vi "SearchAndReplaceJitEx.vi"(4 "Options":u32 format="%.0x", 5 "replace all? (F)":bool, 6 "offset":i32, 7 "substring to replace":i32, 8 "error in":errorcluster, 9 "replace string":string, 10 "search pattern":string, 11 "string":string) -> (0 "error out":errorcluster, 1 "offset past replacement":i32, 2 "number of replacements":i32, 3 "string":string)   [LabVIEW 2021, in "libpcre2-8.lvlib"]
uses:
  libpcre2-8.lvlib
  Pcre2GetOvectorPointer8.vi
  Pcre2MoOfSubstrNumFmOv.vi
  Pcre2SubstringFromSubjectByOffsets (s).vi
  Pcre2CompileError.vi
  Pcre2FnkCallError.vi
  Pcre2ErrorNull.vi
  Pcre2LibError.vi
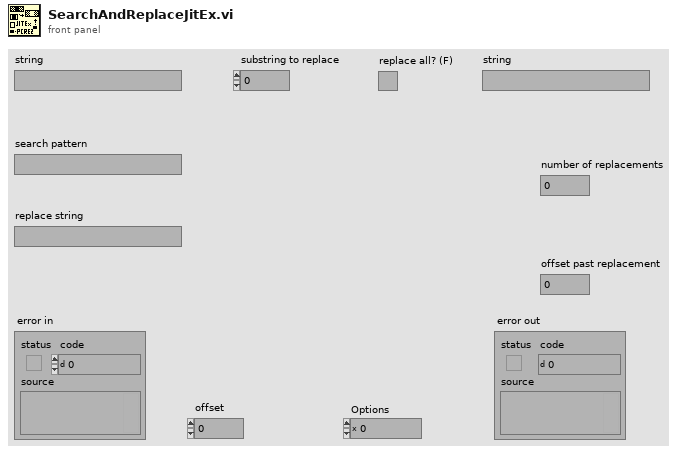
[diagram p1: front panel]
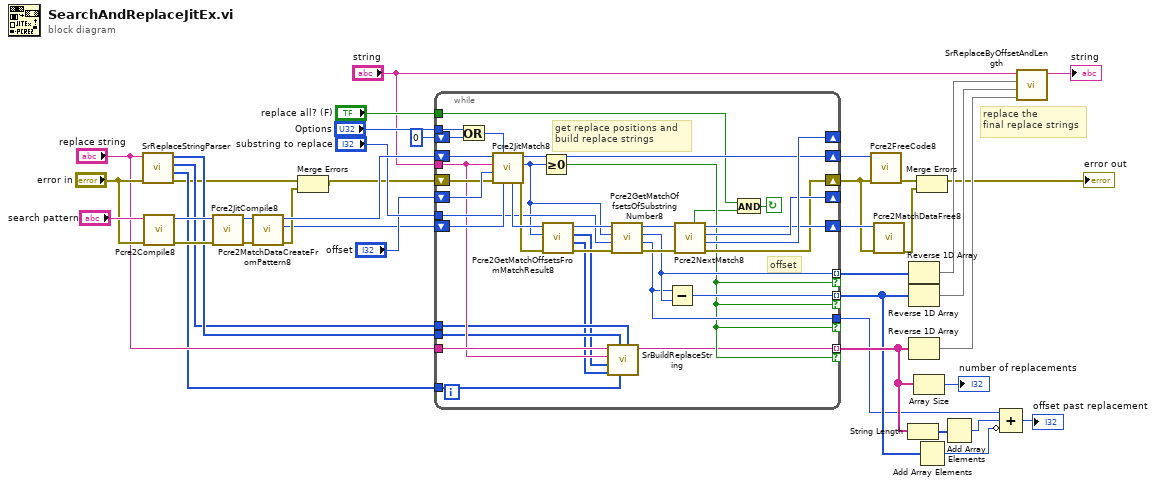
[diagram p0: block diagram]
diagram:
  # "replace the \nfinal replace strings"
  n1 = call "SrReplaceStringParser.vi"("error in"="error in", "ReplaceString"="replace string") -> ("error out"=w5:errorcluster, "ReplSubStrNum"=w14:i32[], "ReplStrLengths"=w15:i32[], "ReplStrOffsets"=w16:i32[])  [unwired: 6 in]
  n2 = call "Pcre2Compile8.vi"("error in"="error in", "Pattern"="search pattern") -> ("error out"=w37:errorcluster, "pCode"=w36:u64)  [unwired: 8 in]
  n3 = call "Pcre2JitCompile8.vi"("error in"=w37, "pCode"=w36) -> ("error out"=w40:errorcluster, "pCode"=w38:u64)  [unwired: 8 in]
  n4 = call "Pcre2MatchDataCreateFromPattern8.vi"("error in"=w40, "pCode"=w38) -> ("error out"=w4:errorcluster, "pMatchData"=w1:u64, "pCode"=w39:u64)  [unwired: 7 in]
  n5 = Merge Errors(w5, w4) -> (w3:errorcluster)
  n6 = while {
    tunnel: "string" -> [w47]
    shift-right: [w71] -> _
    shift-left: "offset" -> [w74]
    shift-right: [w69] -> w32
    shift-left: w1 -> [w73]
    shift-right: [w72] -> _
    shift-left: u32 0 ("GlobalOptions") -> [w56]
    shift-right: [w70] -> w33
    shift-left: w39 -> [w75]
    shift-right: [w67] -> w31
    shift-left: w3 -> [w68]
    tunnel: "replace string" -> [w48]
    tunnel: "substring to replace" -> [w63]
    tunnel: [w41] -> w26 mode=indexing if=w52
    tunnel: [w59] -> w25 mode=indexing if=w52
    tunnel: [w58] -> w34 mode=indexing if=w52
    tunnel: "Options" -> [w54]
    tunnel: [w53] -> w23 if=w52
    tunnel: "replace all? (F)" -> [w51]
    tunnel: w16 -> [w46]
    tunnel: w15 -> [w45]
    tunnel: w14 -> [w44]
    stop <- w49 continue-if-true
    # "get replace positions and \nbuild replace strings"
    # "offset"
    n7 = Or(x=w54, y=w56) -> (x .or. y?=w55:u32)
    n8 = call "Pcre2JitMatch8.vi"("pMatchData"=w73, "Options"=w55, "error in"=w68, "StartOffset"=w74, "Subject"=w47, "pCode"=w75) -> ("error out"=w65:errorcluster, "MatchResult"=w60:i32, "pCode"=w70:u64, "pMatchData"=w66:u64)  [unwired: 2 in]
    n9 = Greater Or Equal To 0?(x=w60) -> (x >= 0?=w52:bool)
    n10 = call "Pcre2GetMatchOffsetsFromMatchResult8.vi"("error in"=w65, "MatchResult"=w60, "pMatchData"=w66) -> ("error out"=w57:errorcluster, "OffsetsPastMatch"=w43:i32[], "MatchOffsets"=w42:i32[], "pMatchData"=w64:u64)  [unwired: 5 in]
    n11 = call "SrBuildReplaceString.vi"("ReplStrLengths"=w45, "ReplSubStrNum"=w44, "ReplStrOffsets"=w46, "OffsetsPastMatch"=w43, "MatchOffsets"=w42, "Subject"=w47, "ReplaceString"=w48) -> ("ReplaceString"=w41:string)  [unwired: 4 in]
    n12 = call "Pcre2GetMatchOffsetsOfSubstringNumber8.vi"("error in"=w57, "Number"=w63, "MatchResult"=w60, "pMatchData"=w64) -> ("error out"=w61:errorcluster, "OffsetPastMatch"=w53:i32, "MatchOffset"=w58:i32, "pMatchData"=w62:u64)  [unwired: 4 in]
    n13 = Subtract(x=w53, y=w58) -> (x-y=w59:i32)
    n14 = call "Pcre2NextMatch8.vi"("error in"=w61, "pMatchData"=w62) -> ("error out"=w67:errorcluster, "GlobalOptions"=w72:u32, "NextStartOffset"=w71:u64, "pMatchData"=w69:u64, "ContinueMatch?"=w50:bool)  [unwired: 5 in]
    n15 = And(x=w51, y=w50) -> (x .and. y?=w49:bool)
  }
  n16 = call "Pcre2FreeCode8.vi"("error in"=w31, "pCode"=w33) -> ("error out"=w7:errorcluster)  [unwired: 9 in]
  n17 = call "Pcre2MatchDataFree8.vi"("error in"=w31, "pMatchData"=w32) -> ("error out"=w6:errorcluster)  [unwired: 9 in]
  n18 = String Length(string=w26) -> (length=w24:i32[])
  n19 = Reverse 1D Array(array=w34) -> (reversed array=w11:i32[])
  n20 = Reverse 1D Array(array=w25) -> (reversed array=w10:i32[])
  n21 = Reverse 1D Array(array=w26) -> (reversed array=w9:string[])
  n22 = Array Size(array=w26) -> (size(s)=→"number of replacements":i32)
  n23 = Merge Errors(w7, w6) -> (→"error out":errorcluster)
  n24 = Add Array Elements(numeric array=w25) -> (sum=w22:i32)
  n25 = Add Array Elements(numeric array=w24) -> (sum=w20:i32)
  n26 = Compound Arithmetic op=ADD(w23, w20, invert w22) -> (→"offset past replacement":i32)
  n27 = call "SrReplaceByOffsetAndLength.vi"("Replace"=w9, "Lengths"=w10, "Offsets"=w11, "String"="string") -> ("String"=→"string":string)  [unwired: 7 in]
